vi "2ALABVIEW.vi"() -> ()   [LabVIEW 2013]
panel:
  out "OUTPUT":dbl
  in  "B":dbl
  in  "A":dbl
  # "SUM OF 'n' NUMBERS USING FOR LOOP"
  # "O.SRINIVAS\n23A91A04H6"
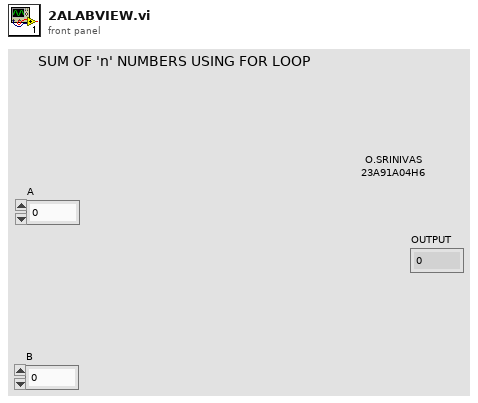
[diagram p1: front panel]
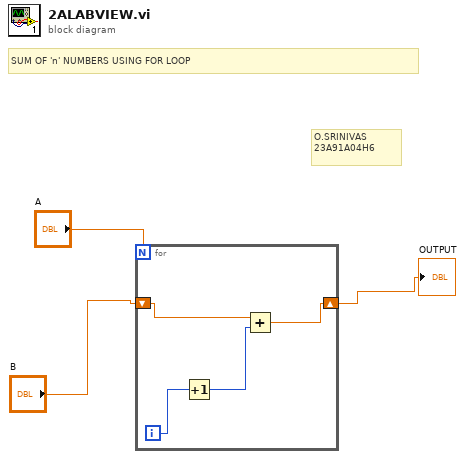
[diagram p0: block diagram]
diagram:
  # "SUM OF 'n' NUMBERS USING FOR LOOP"
  # "O.SRINIVAS\n23A91A04H6"
  n1 = for {
    N: "A" -> [_]
    shift-right: [w5] -> w2
    shift-left: "B" -> [w4]
    i -> [w6]
    n2 = Increment(x=w6) -> (x+1=w7:i32)
    n3 = Add(x=w4, y=w7) -> (x+y=w5:dbl)
  }
  "OUTPUT" <- w2
